vi "ReportError.vi"(8 "error in (no error)":errorcluster, 10 "ErrorReported":errorcluster, 11 "ModuleID":i32) -> (0 "error out":errorcluster)   [LabVIEW 2018, in "AcPwrPlugins.lvlib"]
doc: "This VI broadcasts any error that occurs in Main.vi."
uses:
  AcPwrPlugins.lvlib
  AcPwrShared/clEventType.ctl
  AcPwrShared/AcPwrShared.lvlib
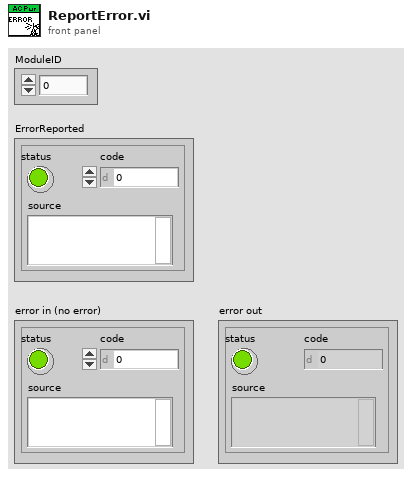
[diagram p1: front panel]
types:
  T1 = typedef "AcPwrShared.lvlib/clEventType.ctl" = cluster{"ModuleID":i32, "Data":variant}
  T2 = typedef "AcPwrShared.lvlib/clBroadcastEvents.ctl" = cluster{"DidInit":refnum<user-event>, "StatusUpdate":refnum<user-event>, "ErrorReport":refnum<user-event>, "DidStop":refnum<user-event>, "PathToINI":refnum<user-event>, "Measurements":refnum<user-event>, "LoadConfigFile":refnum<user-event>, "GetSettings":refnum<user-event>, "SetSettings":refnum<user-event>, "GetType&ID":refnum<user-event>, "GotSettings":refnum<user-event>}
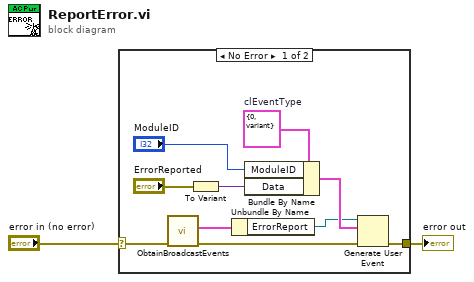
[diagram p0: block diagram]
diagram:
  n1 = case shown="No Error" "error in (no error)" {
    selector: "error in (no error)" -> [w4 w13]
    tunnel: [w5 w13] -> w1
    frame No Error {
      w12 = T1 {"ModuleID"=0, "Data"=variant}  # clEventType
      n2 = call "ObtainBroadcastEvents.vi"("error in (no error)"=w4) -> ("error out"=w3:errorcluster, "clAcPwrEvents"=w9:T2)  [unwired: 9 in]
      n3 = To Variant(anything="ErrorReported") -> (Variant=w11:variant)
      n4 = Unbundle By Name(w9) -> ("ErrorReport"=w7:refnum<user-event>)
      n5 = Bundle By Name(cluster=w12, "ModuleID"="ModuleID", "Data"=w11) -> (w8:T1)
      n6 = Generate User Event(user event=w7, event data cluster=w8, error in=w3) -> (error out=w5:errorcluster)  [unwired: 1 in, 1 out]
    }
    frame Error {
    }
  }
  "error out" <- w1
